vi "Is Naughty SubVI.vi"(7 "Disallowed SubVI Paths":string[](array[string]), 10 "GObj Refnum":refnum<vi>) -> (1 "SubVI":string, 2 "Naughty SubVI":bool, 3 "VIPath":path, 4 "Missing SubVI":bool, 5 "Is SubVI":bool)   [LabVIEW 2020, in "SoL Inspector.lvlib"]
uses:
  SoL Inspector.lvlib
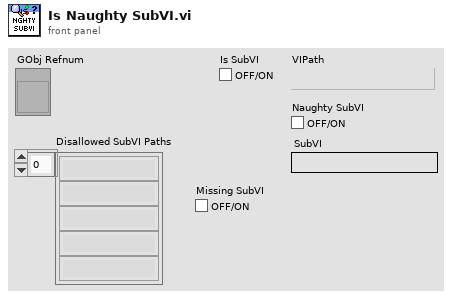
[diagram p1: front panel]
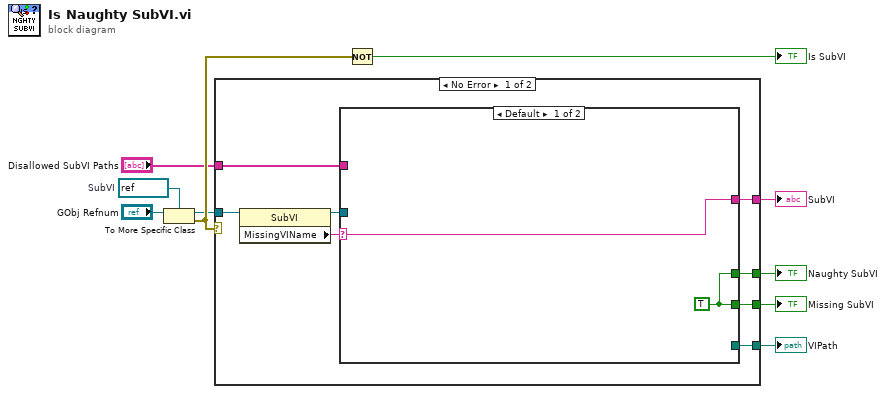
[diagram p0: block diagram]
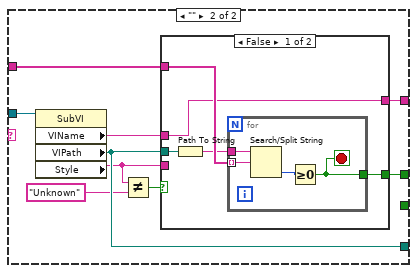
[diagram p2: hidden frame]
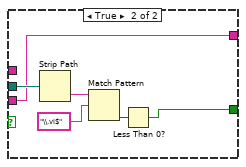
[diagram p3: hidden frame]
diagram:
  w8 = refnum<vi> refnum  # SubVI
  n1 = To More Specific Class(target class=w8, reference="GObj Refnum") -> (specific class reference=w7:refnum<vi>, error out=w10:errorcluster)  [unwired: 1 in]
  n2 = case shown="No Error" w10 {
    tunnel: w7 -> [w14 _]
    tunnel: [w18 _] -> w6
    tunnel: [w15 _] -> w5
    tunnel: [w17 _] -> w4
    tunnel: "Disallowed SubVI Paths" -> [w16 _]
    tunnel: [w11 _] -> w2
    frame No Error {
      n3 = property class="SubVI"(reference=w14) -> (reference out=w13:refnum<vi>, "MissingVIName"=w12:string)  [unwired: 1 in, 1 out]
      n4 = case shown="Default" w12 {
        selector: w12 -> [w19 _]
        tunnel: [w20 w29] -> w18
        tunnel: [_ w28] -> w17
        tunnel: w16 -> [_ w27]
        tunnel: [w19 w22] -> w15
        tunnel: w13 -> [_ w21]
        tunnel: [w20 _] -> w11
        frame Default {
          w20 = TRUE
        }
        frame "" {
          n5 = property class="SubVI"(reference=w21) -> ("VIName"=w24:string, "VIPath"=w28:path, "Style"=w23:string)  [unwired: 1 in, 2 out]
          n6 = Not Equal?(x=w23, y="Unknown") -> (x != y?=w25:bool)
          n7 = case shown="False" w25 {
            tunnel: [w34 w40] -> w29
            tunnel: w28 -> [w33 w42]
            tunnel: w27 -> [w32 _]
            tunnel: w24 -> [w30 _]
            tunnel: w23 -> [_ w39]
            tunnel: [w30 w39] -> w22
            frame False {
              n8 = Path To String(path=w33) -> (string=w31:string)
              n9 = for {
                tunnel: w31 -> [w37]
                tunnel: [w38] -> w34
                tunnel: w32 -> [w36] mode=indexing
                stop <- w38 stop-if-true
                n10 = Search/Split String(string=w37, search string/char (-)=w36) -> (offset of match=w35:i32)  [unwired: 1 in, 2 out]
                n11 = Greater Or Equal To 0?(x=w35) -> (x >= 0?=w38:bool)
              }
            }
            frame True {
              n12 = Strip Path(path=w42) -> (name=w41:string)  [unwired: 1 out]
              n13 = Match Pattern(string=w41, regular expression="\\.vi$") -> (offset past match=w43:i32)  [unwired: 1 in, 3 out]
              n14 = Less Than 0?(x=w43) -> (x < 0?=w40:bool)
            }
          }
        }
      }
    }
    frame Error {
    }
  }
  "Naughty SubVI" <- w6
  "SubVI" <- w5
  "VIPath" <- w4
  "Missing SubVI" <- w2
  n15 = Not(x=w10) -> (.not. x?=→"Is SubVI":bool)
